vi "GEA2 Flash APL.vi"(0 "GEA2 Reference In":refnum<k24>, 2 "Force Update?":bool, 5 "Source Address":u8=228 format="%.0x", 7 "Destination Address":u8 format="%.0x", 9 "File Path":path, 11 "Error In":errorcluster, 12 "Broadcast":bool=TRUE, 13 "Reset?":bool=TRUE) -> (4 "GEA2 Reference Out":refnum<k24>, 6 "Result":i32(ring) items=["InvalidImage", "ImageRejected", "BoardNotFound", "UnableToGetGeaConfiguration", "WriteToFlashNotAllowed", "ImageDownloadedSuccessfully", "ImagePresent", "WriteToFlashFailed", "EraseFailed", "CrcFailed"], 8 "Pass/Fail":bool, 10 "Report Text":string, 15 "Error Out":errorcluster)   [LabVIEW 2014, in "GEA2_Toolkit.lvlib"]
doc: "This VI will flash an APL file onto an appliance board. The input 'Filename' accepts a string with file extension, for example 'MC_v1.06.apl'. Force Update will ensure the APL is downloaded even if it is the same version as what already exists on the appliance board."
uses:
  library/GEA2_Toolkit.lvlib
  C:/Automation/DLLs/PC Tools .NET/Programming.dll
  Automation/DLLs/PC Tools .NET/Programming.dll
  C:/Automation/DLLs/PC Tools .NET/GeaCommunication.dll
  Automation/DLLs/PC Tools .NET/GeaCommunication.dll
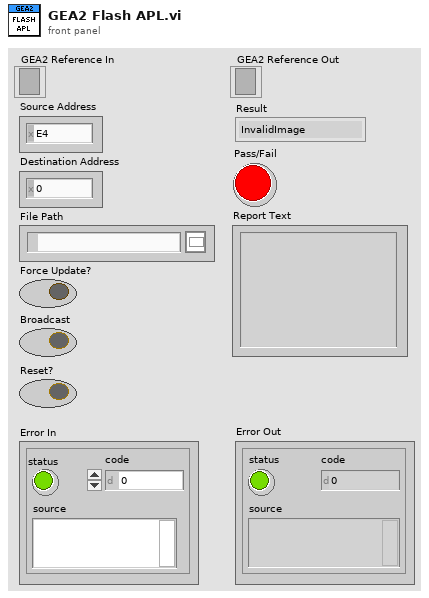
[diagram p1: front panel]
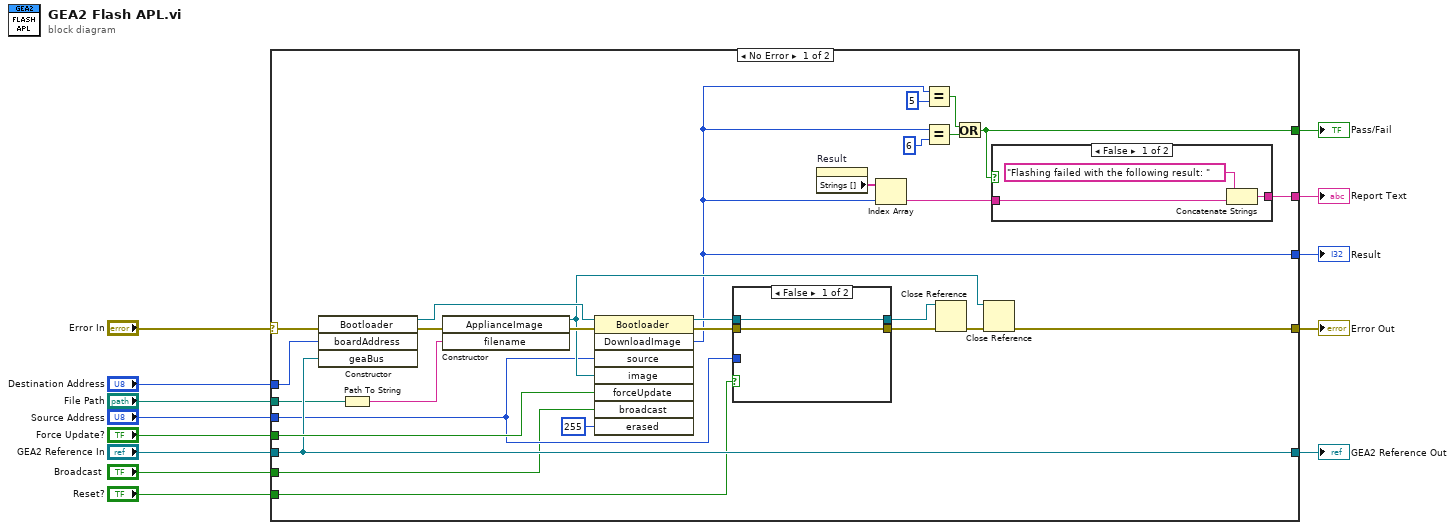
[diagram p0: block diagram]
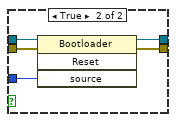
[diagram p2: hidden frame]
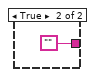
[diagram p3: hidden frame]
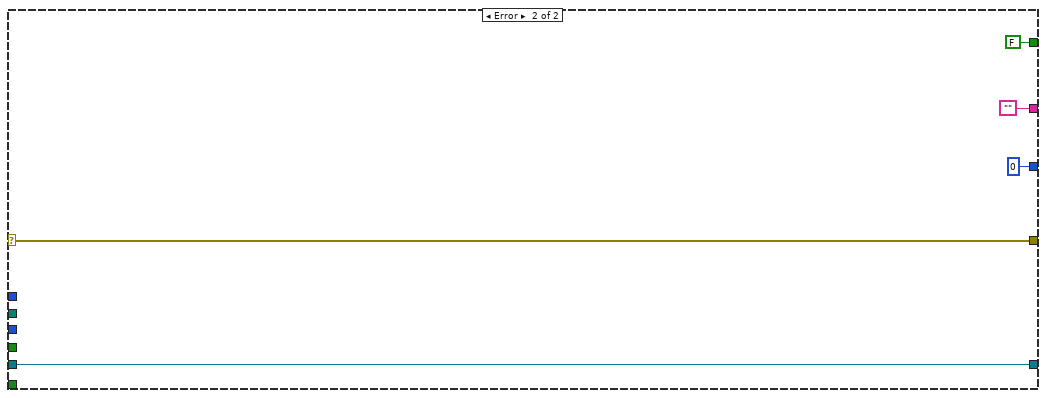
[diagram p4: hidden frame]
diagram:
  n1 = case shown="No Error" "Error In" {
    selector: "Error In" -> [w33 w57]
    tunnel: "GEA2 Reference In" -> [w32 w58]
    tunnel: "Destination Address" -> [w42 _]
    tunnel: "Force Update?" -> [w40 _]
    tunnel: "Source Address" -> [w27 _]
    tunnel: [w19 0 ("DownloadImage")] -> w9
    tunnel: [w34 w57] -> w8
    tunnel: [w32 w58] -> w6
    tunnel: "File Path" -> [w25 _]
    tunnel: "Broadcast" -> [w24 _]
    tunnel: [w18 FALSE] -> w3
    tunnel: [w16 ""] -> w2
    tunnel: "Reset?" -> [w14 _]
    frame No Error {
      n2 = constructor class="Bootloader"(error in=w33, "boardAddress"=w42, "geaBus"=w32) -> (reference out=w38:refnum<k24>, error out=w41:errorcluster)  [unwired: 2 in, 3 out]
      n3 = Path To String(path=w25) -> (string=w26:string)
      n4 = constructor class="ApplianceImage"(error in=w41, "filename"=w26) -> (reference out=w36:refnum<k24>, error out=w39:errorcluster)  [unwired: 2 in, 2 out]
      n5 = invoke class="Bootloader" method="DownloadImage"(reference=w38, error in=w39, "source"=w27, "image"=w36, "forceUpdate"=w40, "broadcast"=w24, "erased"=u8 255) -> (reference out=w31:refnum<k24>, error out=w30:errorcluster, "DownloadImage"=w19:i32)  [unwired: 1 in, 5 out]
      n6 = case shown="False" w14 {
        tunnel: w31 -> [w43 w49]
        tunnel: w30 -> [w44 w48]
        tunnel: [w43 w47] -> w29
        tunnel: [w44 w46] -> w28
        tunnel: w27 -> [_ w45]
        frame False {
        }
        frame True {
          n7 = invoke class="Bootloader" method="Reset"(reference=w49, error in=w48, "source"=w45) -> (reference out=w47:refnum<k24>, error out=w46:errorcluster)  [unwired: 1 in, 2 out]
        }
      }
      n8 = property on="Result" class="Ring (strict)"() -> ("Strings []"=w15:string[])  [unwired: 2 in, 2 out]
      n9 = Index Array(array=w15, index=w19) -> (element=w17:string)
      n10 = Equal?(x=w19, y=5) -> (x = y?=w22:bool)
      n11 = Equal?(x=w19, y=6) -> (x = y?=w23:bool)
      n12 = Close Reference(reference=w29, error in (no error)=w28) -> (error out=w37:errorcluster)
      n13 = Or(x=w22, y=w23) -> (x .or. y?=w18:bool)
      n14 = Close Reference(reference=w36, error in (no error)=w37) -> (error out=w34:errorcluster)
      n15 = case shown="False" w18 {
        tunnel: w17 -> [w51 _]
        tunnel: [w50 ""] -> w16
        frame False {
          n16 = Concatenate Strings("Flashing failed with the following result: ", w51) -> (w50:string)
        }
        frame True {
        }
      }
    }
    frame Error {
    }
  }
  "GEA2 Reference Out" <- w6
  "Result" <- w9
  "Error Out" <- w8
  "Pass/Fail" <- w3
  "Report Text" <- w2
